vi "FPGA_Read.vi"(6 "Espera acceso USB":u32=20, 8 "error in":errorcluster, 9 "Numero Bytes":u8, 10 "Dirección base":u8, 11 "ftHandle_in":u32) -> (0 "error out":errorcluster, 1 "lpBytesWritten":u32=44, 2 "lpBuffer_out":u8[](array[numeric])=[1, 0, 0, 0, 184, 0, 16, 224, 0, 2, 113, 76, 75, 64, 0, 0, 39, 0, 24, 52, 33, 241, 29, 50, 41, 102, 53, 71, 78, 101, 89, 183, 105, 43, 121, 27, 136, 207, 144, 0, 160, 0, 176, 0] format="%.0x", 3 "ftHandle_out":u32=318917776, 4 "status":u32)   [LabVIEW 2019]
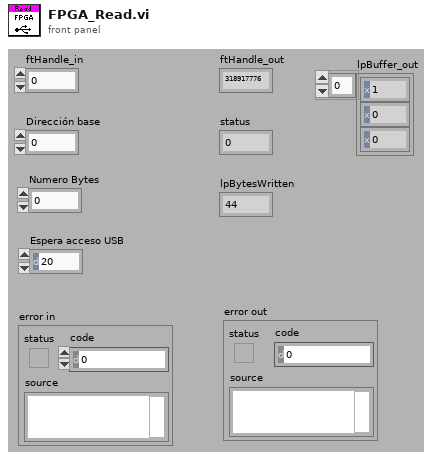
[diagram p1: front panel]
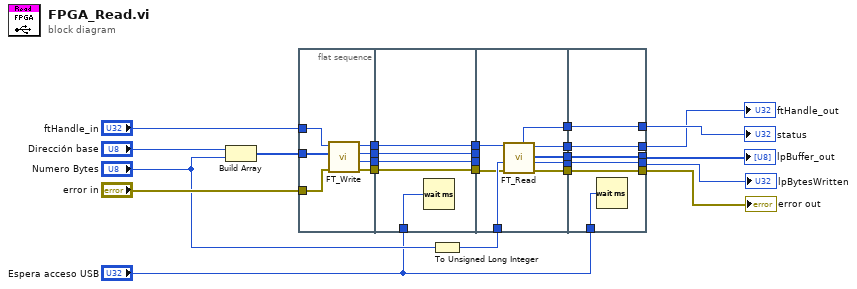
[diagram p0: block diagram]
diagram:
  n1 = Build Array("Dirección base", "Numero Bytes") -> (w18:u8[])
  n2 = flat-sequence {
    tunnel: "error in" -> [w32]
    tunnel: "ftHandle_in" -> [w28]
    tunnel: w18 -> [w27]
    tunnel: [w31] -> w17
    tunnel: [w26] -> w16
    tunnel: [w30] -> w15
    tunnel: [w29] -> w14
    tunnel: w17 -> [w37]
    tunnel: w16 -> [w36]
    tunnel: w15 -> [w35]
    tunnel: w14 -> [w34]
    tunnel: [w37] -> w13
    tunnel: [w36] -> w12
    tunnel: [w35] -> w11
    tunnel: [w34] -> w10
    tunnel: "Espera acceso USB" -> [w33]
    tunnel: w13 -> [_]
    tunnel: w12 -> [_]
    tunnel: w11 -> [w41]
    tunnel: w10 -> [w45]
    tunnel: w8 -> [w42]
    tunnel: [w39] -> w6
    tunnel: [w43] -> w5
    tunnel: [w40] -> w4
    tunnel: [w44] -> w3
    tunnel: [w38] -> w2
    tunnel: [w47] -> w7
    tunnel: [w48] -> w21
    tunnel: [w49] -> w22
    tunnel: [w50] -> w23
    tunnel: [w51] -> w24
    tunnel: w6 -> [w51]
    tunnel: w5 -> [w50]
    tunnel: w4 -> [w49]
    tunnel: w3 -> [w48]
    tunnel: w2 -> [w47]
    tunnel: "Espera acceso USB" -> [w46]
    frame #0 {
      n3 = call "FT_Write.vi"("error in (no error)"=w32, "lpBuffer"=w27, "ftHandle_in"=w28) -> ("error out"=w30:errorcluster, "lpBytesWritten"=w31:u32, "status"=w26:u32, "ftHandle_out"=w29:u32)  [unwired: 5 out]
    }
    frame #1 {
      n4 = Wait (ms)(milliseconds to wait=w33) -> ()  [unwired: 1 out]
    }
    frame #2 {
      n5 = call "FT_Read.vi"("error in (no error)"=w41, "dwBytestoRead"=w42, "ftHandle_in"=w45) -> ("error out"=w40:errorcluster, "lpBytesReturned"=w39:u32, "lpBuffer_out"=w38:u8[], "ftHandle_out"=w44:u32, "status"=w43:u32)  [unwired: 4 out]
    }
    frame #3 {
      n6 = Wait (ms)(milliseconds to wait=w46) -> ()  [unwired: 1 out]
    }
  }
  n7 = To Unsigned Long Integer(number="Numero Bytes") -> (unsigned 32bit integer=w8:u32)
  "lpBytesWritten" <- w24
  "status" <- w23
  "error out" <- w22
  "ftHandle_out" <- w21
  "lpBuffer_out" <- w7
